vi "daqReadEtlSegment.vi"() -> ()   [LabVIEW 2017]
doc: "From the DAQ card, reads into shared variables the external frame counter, the piezo monitor, and its differentiator. The acquisition is triggered by the Hamamatsu camera triggers. If daqSave is set to true, writes the values to file. \n\nThe acquisition loop stops with a daqStop (generally issued by the hamamatsuRead* VI) or, after a delay, with a generalStop."
uses:
  <vilib>/DAQmx/read.llb/DAQmx Read (Analog 1D DBL NChan 1Samp).vi
  <vilib>/DAQmx/read.llb/DAQmx Read (Digital Bool 1Line 1Point).vi
  <vilib>/DAQmx/read.llb/DAQmx Read (Counter U32 1Chan 1Samp).vi
  globalDevices.vi
  globalUtilities.vi
  <vilib>/DAQmx/miscellaneous.llb/DAQmx Fill In Error Info.vi
panel:
  out "#problems with frame cntr":u32
  out "problem with frame counter":bool
  out "data":bool
  out "success":bool
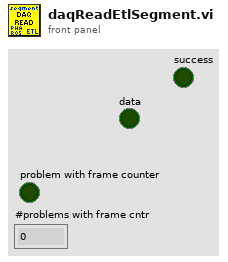
[diagram p1: front panel]
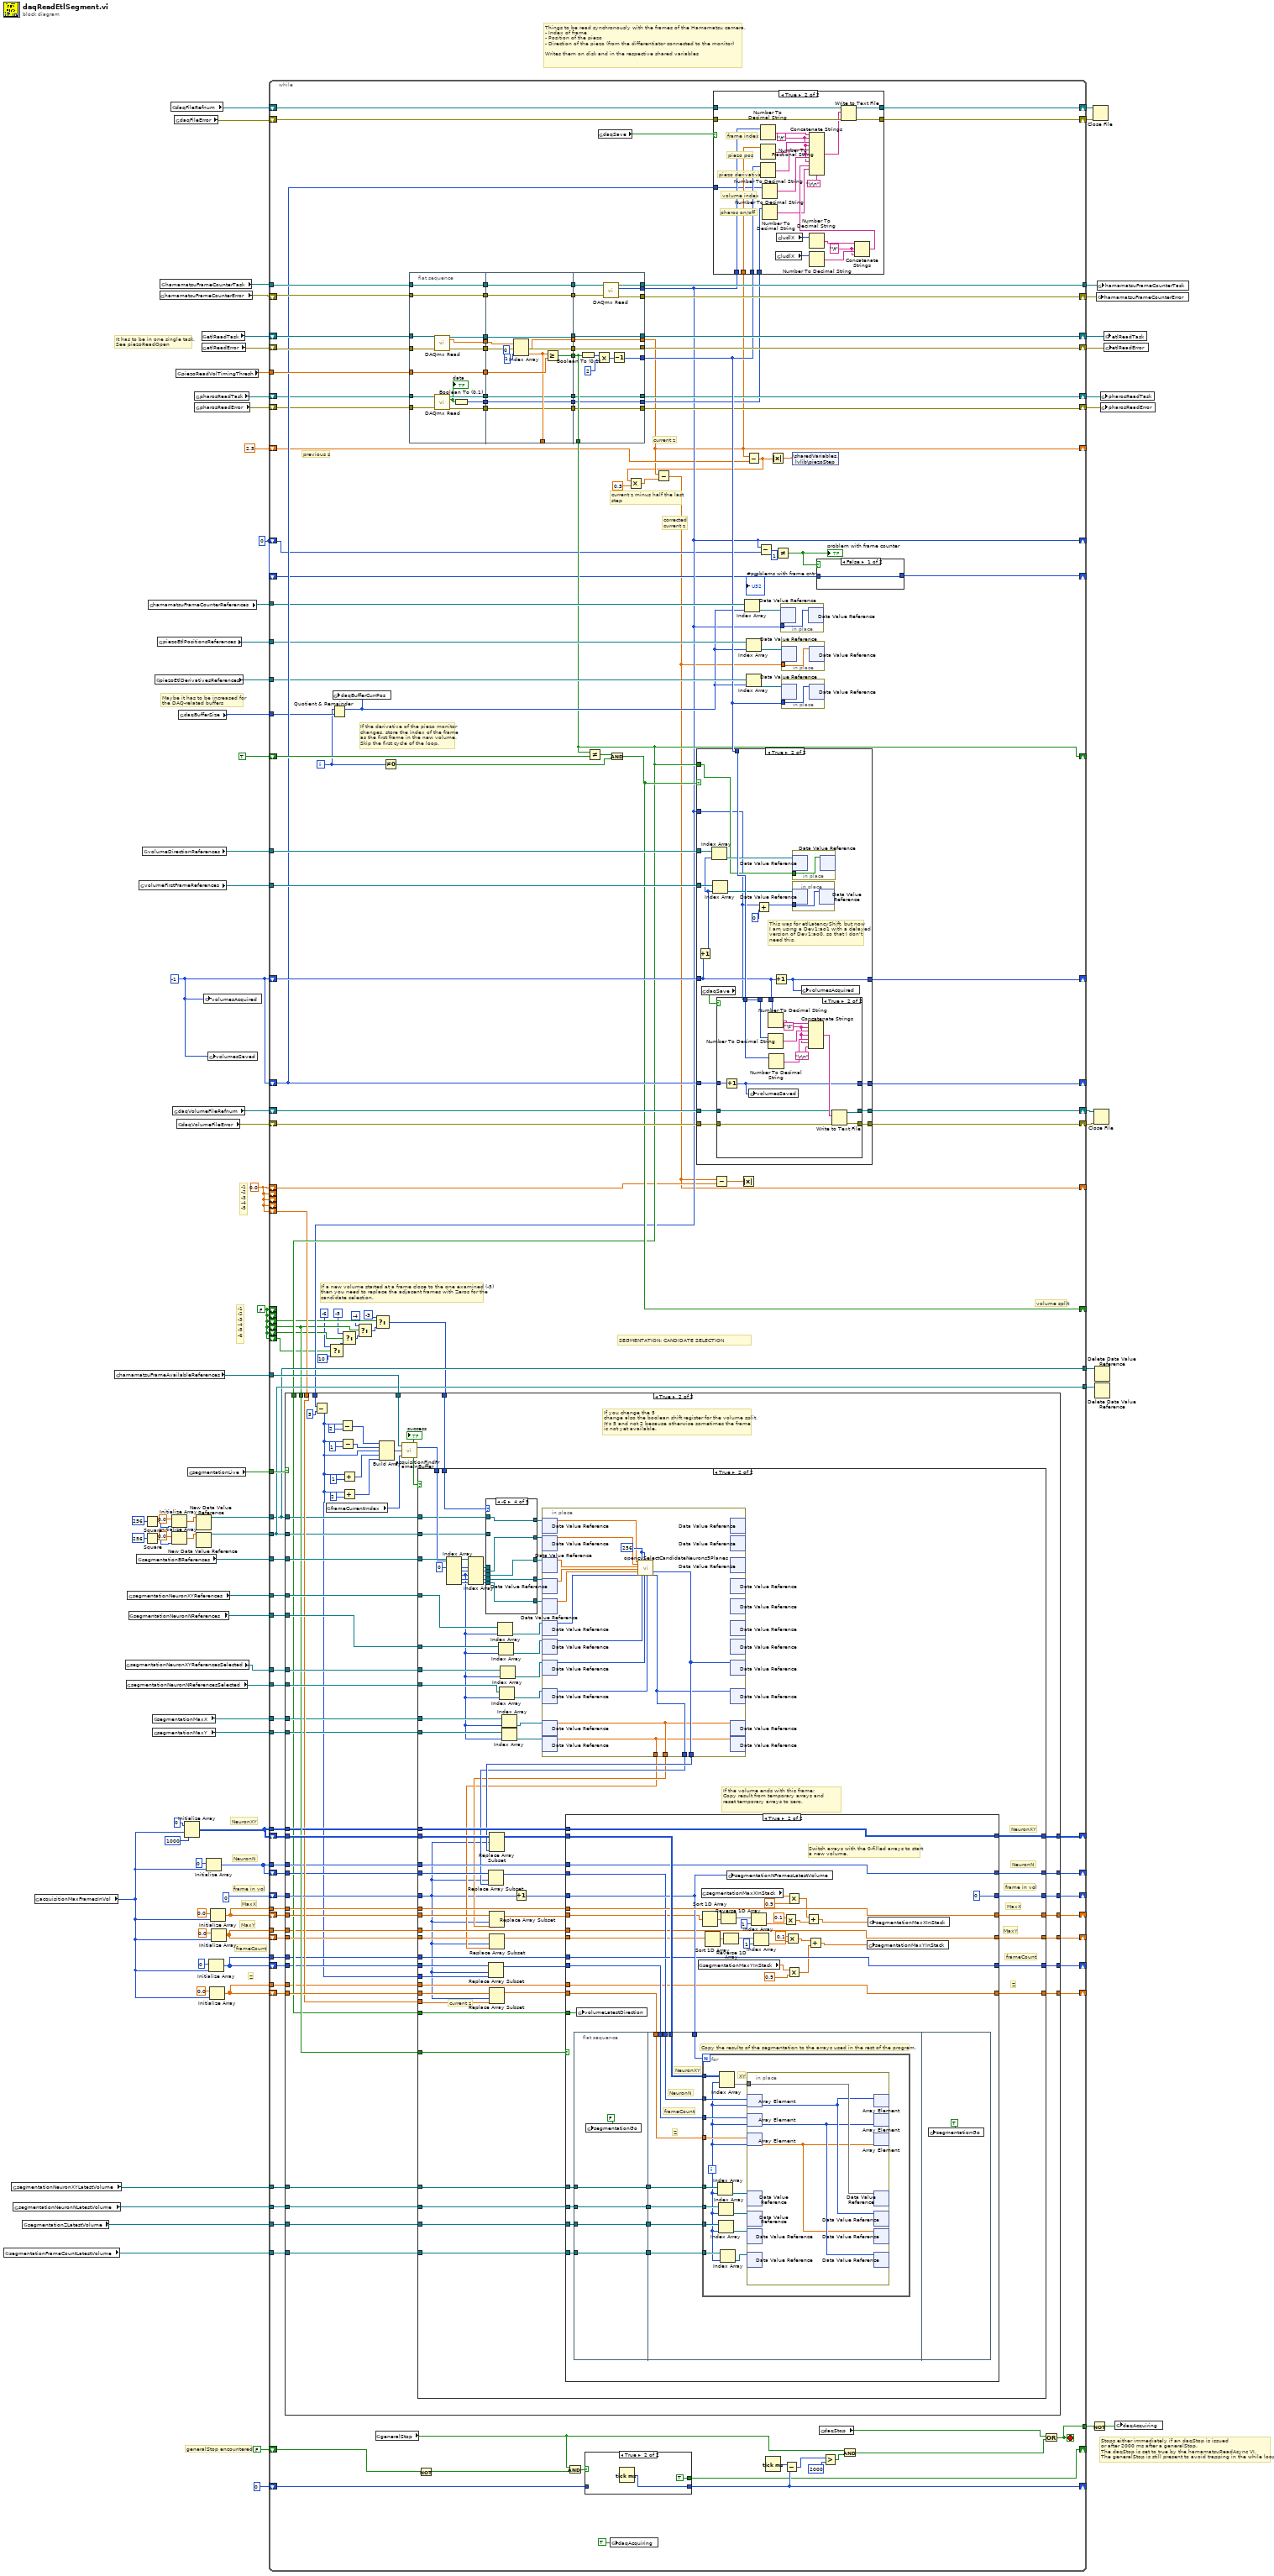
[diagram p0: block diagram]
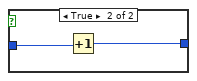
[diagram p2: hidden frame]
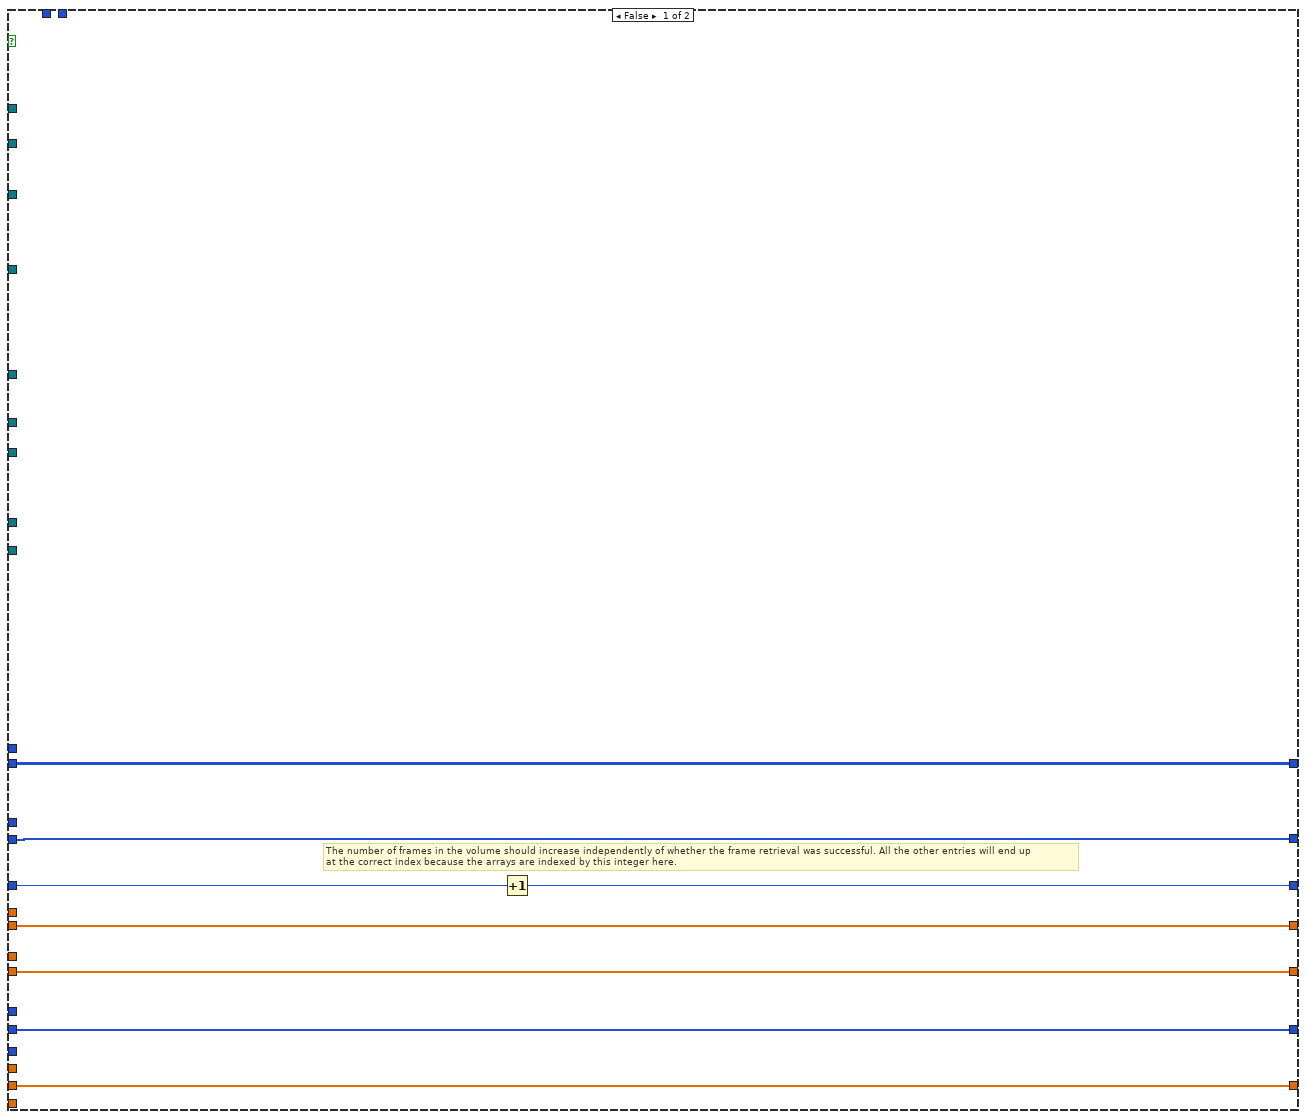
[diagram p4: hidden frame]
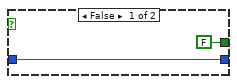
[diagram p12: hidden frame]
diagram:
  w9 = u32 0 ("data")
  w4 = FALSE
  w55 = -1
  w14 = 0.0
  # "Z"
  # "frameCount"
  # "MaxY"
  # "MaxX"
  # "frame in vol"
  # "NeuronN"
  # "NeuronXY"
  # "-1\n-2\n-3\n-4\n-5"
  # "-1\n-2\n-3\n-4\n-5\n-6"
  # "Maybe it has to be increased for\nthe DAQ-related buffers"
  # "It has to be in one single task.\nSee piezoReadOpen"
  # "generalStop encountered"
  # "Stops either immediately if an daqStop is issued\nor after 2000 ms after a generalStop.\nThe daqStop is set to true by the hamamatsuReadAsync VI.\nThe generalStop is still present to avoid trapping in the while loop."
  # "Things to be read synchronously with the frames of the Hamamatsu camera.\n- Index of frame\n- Position of the piezo\n- Direction of the piezo (from the differentiator connected to the monitor)\n\nWrites them on disk and in the respective shared variables"
  n1 = global read "globalUtilities.vi" "segmentationFrameCountLatestVolume"() -> (w8:refnum<data-value>[])
  n2 = global read "globalUtilities.vi" "segmentationNeuronXYLatestVolume"() -> (w37:refnum<data-value>[])
  n3 = global read "globalUtilities.vi" "segmentationNeuronNLatestVolume"() -> (w36:refnum<data-value>[])
  n4 = global read "globalUtilities.vi" "segmentationZLatestVolume"() -> (w33:refnum<data-value>[])
  n5 = global read "globalUtilities.vi" "acquisitionMaxFramesInVol"() -> (w6:i32)
  n6 = global read "globalDevices.vi" "hamamatsuFrameAvailableReferences"() -> (w42:refnum<data-value>[])
  n7 = global read "globalUtilities.vi" "segmentationNeuronXYReferencesSelected"() -> (w44:refnum<data-value>[])
  n8 = global read "globalUtilities.vi" "segmentationNeuronNReferencesSelected"() -> (w43:refnum<data-value>[])
  n9 = global read "globalUtilities.vi" "segmentationNeuronXYReferences"() -> (w45:refnum<data-value>[])
  n10 = global read "globalUtilities.vi" "segmentationNeuronNReferences"() -> (w47:refnum<data-value>[])
  n11 = global read "globalUtilities.vi" "segmentationBReferences"() -> (w48:refnum<data-value>[])
  n12 = global read "globalUtilities.vi" "volumeFirstFrameReferences"() -> (w56:refnum<data-value>[])
  n13 = global read "globalUtilities.vi" "volumeDirectionReferences"() -> (w57:refnum<data-value>[])
  n14 = Square(x=256) -> (x^2=w18:i32)
  n15 = Square(x=256) -> (x^2=w31:i32)
  n16 = global read "globalDevices.vi" "hamamatsuFrameCounterReferences"() -> (w52:refnum<data-value>[])
  n17 = global read "globalUtilities.vi" "segmentationMaxX"() -> (w26:refnum<data-value>[])
  n18 = global read "globalUtilities.vi" "segmentationMaxY"() -> (w25:refnum<data-value>[])
  n19 = global read "globalDevices.vi" "piezoEtlDerivativesReferences"() -> (w50:refnum<data-value>[])
  n20 = global read "globalDevices.vi" "piezoEtlPositionsReferences"() -> (w51:refnum<data-value>[])
  n21 = global read "globalDevices.vi" "hamamatsuFrameCounterError"() -> (w76:errorcluster)
  n22 = global read "globalDevices.vi" "hamamatsuFrameCounterTask"() -> (w77:refnum<k21>)
  n23 = global read "globalDevices.vi" "daqFileRefnum"() -> (w66:refnum<file>)
  n24 = Initialize Array(sgl 0.0 ("element"), w18) -> (w17:sgl[])
  n25 = Initialize Array(sgl 0.0 ("element"), w31) -> (w32:sgl[])
  n26 = global read "globalDevices.vi" "daqVolumeFileRefnum"() -> (w61:refnum<file>)
  n27 = global read "globalDevices.vi" "daqFileError"() -> (w65:errorcluster)
  n28 = global read "globalDevices.vi" "piezoReadVolTimingThresh"() -> (w72:dbl)
  n29 = global read "globalDevices.vi" "daqVolumeFileError"() -> (w60:errorcluster)
  n30 = global read "globalDevices.vi" "daqBufferSize"() -> (w49:i32)
  n31 = Initialize Array(u16 0 ("element"), w6, 1000 ("dimension size")) -> (w35:u16[][])
  n32 = global read "globalUtilities.vi" "segmentationLive"() -> (w46:bool)
  n33 = global read "globalDevices.vi" "pharosReadTask"() -> (w13:refnum<k21>)
  n34 = global read "globalDevices.vi" "pharosReadError"() -> (w12:errorcluster)
  n35 = New Data Value Reference(data value=w17) -> (data value reference=w16:refnum<data-value>)  [unwired: 1 in, 1 out]
  n36 = New Data Value Reference(data value=w32) -> (data value reference=w28:refnum<data-value>)  [unwired: 1 in, 1 out]
  n37 = global read "globalDevices.vi" "etlReadTask"() -> (w54:refnum<k21>)
  n38 = global read "globalDevices.vi" "etlReadError"() -> (w53:errorcluster)
  n39 = global write "globalUtilities.vi" "volumesAcquired"(w55) -> ()
  n40 = Initialize Array(u16 0 ("element"), w6) -> (w21:u16[])
  n41 = global write "globalUtilities.vi" "volumesSaved"(w55) -> ()
  n42 = Initialize Array(0 ("element"), w6) -> (w5:i32[])
  n43 = Initialize Array(0.0 ("element"), w6) -> (w2:dbl[])
  n44 = Initialize Array(0.0 ("element"), w6) -> (w22:dbl[])
  n45 = Initialize Array(0.0 ("element"), w6) -> (w3:dbl[])
  n46 = while {
    tunnel: w77 -> [w217]
    shift-right: [w213] -> w68
    shift-left: w76 -> [w215]
    shift-right: [w211] -> w69
    shift-left: w53 -> [w214]
    shift-right: [w208] -> w75
    shift-left: w66 -> [w209]
    shift-right: [w195] -> _
    shift-left: FALSE -> [w206]
    shift-right: [w200] -> _
    shift-left: u32 0 -> [w203]
    tunnel: w72 -> [w194]
    shift-right: [w126] -> _
    shift-left: TRUE -> [w192]
    shift-right: [w188] -> w70
    shift-left: w54 -> [w219]
    tunnel: [w187] -> w67
    shift-right: [w179] -> w64
    shift-left: w65 -> [w210]
    tunnel: [w176] -> w63
    shift-right: [w82] -> _
    shift-left: w14 -> [w87]
    shift-right: [w172] -> w58
    shift-left: w60 -> [w174]
    shift-right: [w173] -> w59
    shift-left: w61 -> [w175]
    shift-right: [w170] -> _
    shift-left: w55 -> [w171]
    tunnel: w57 -> [w169]
    tunnel: w56 -> [w168]
    shift-right: [w167] -> _
    shift-left: w55 -> [w166]
    tunnel: w52 -> [w165]
    tunnel: w51 -> [w164]
    tunnel: w50 -> [w163]
    tunnel: w49 -> [w162]
    tunnel: w48 -> [w156]
    tunnel: w47 -> [w155]
    tunnel: w46 -> [w150]
    tunnel: w45 -> [w154]
    tunnel: w44 -> [w153]
    tunnel: w43 -> [w152]
    tunnel: w42 -> [w151]
    shift-right: [w147] -> _
    shift-left: w35 -> [w149]
    shift-right: [w148] -> _
    shift-left: w4 -> [_]
    shift-left: w4 -> [_]
    shift-left: w4 -> [w102]
    shift-left: w4 -> [w99]
    shift-left: w4 -> [w97]
    shift-right: [w145] -> _
    shift-left: w21 -> [w146]
    shift-right: [w143] -> _
    shift-left: 0 -> [w144]
    tunnel: w37 -> [w142]
    tunnel: w36 -> [w141]
    tunnel: w35 -> [w140]
    shift-right: [w138] -> _
    shift-left: w2 -> [w139]
    tunnel: w33 -> [w137]
    shift-left: w14 -> [_]
    shift-left: w14 -> [_]
    shift-left: w14 -> [_]
    shift-left: w14 -> [w103]
    tunnel: w28 -> [w136]
    tunnel: [w136] -> w27
    tunnel: w26 -> [w135]
    tunnel: w25 -> [w134]
    shift-right: [w131] -> _
    shift-left: w3 -> [w132]
    shift-right: [w130] -> _
    shift-left: w22 -> [w133]
    tunnel: w22 -> [w129]
    tunnel: w21 -> [w128]
    tunnel: w16 -> [w127]
    tunnel: [w127] -> w15
    shift-right: [w121] -> w11
    shift-left: w13 -> [w125]
    shift-right: [w118] -> w10
    shift-left: w12 -> [w124]
    shift-right: [w114] -> _
    shift-left: w9 -> [w113]
    shift-right: [w109] -> _
    shift-left: w9 -> [w108]
    shift-right: [w106] -> _
    shift-left: w5 -> [w107]
    tunnel: w5 -> [w105]
    tunnel: w8 -> [w104]
    shift-left: w4 -> [w94]
    tunnel: w3 -> [w90]
    tunnel: w2 -> [w89]
    shift-right: [w83] -> _
    shift-left: 2.5 ("Waveform") -> [w84]
    i -> [w85]
    stop <- w176 stop-if-true
    # "corrected\ncurrent z"
    # "current z"
    # "current z minus half the last\nstep"
    # "previous z"
    # "volume split"
    # "SEGMENTATION: CANDIDATE SELECTION"
    # "If a new volume started at a frame close to the one examined (-5)\nthen you need to replace the adjacent frames with Zeros for the\ncandidate selection."
    # "If the derivative of the piezo monitor\nchanges, store the index of the frame\nas the first frame in the new volume.\nSkip the first cycle of the loop."
    n47 = Select(t=-6, s=w94, f=10) -> (s? t:f=w92:i32)
    n48 = Quotient & Remainder(x=w85, y=w162) -> (x-y*floor(x/y)=w157:i32)  [unwired: 1 out]
    n49 = global write "globalDevices.vi" "daqBufferCurrPos"(w157) -> ()
    n50 = Select(t=-5, s=w97, f=w92) -> (s? t:f=w95:i32)
    n51 = Select(t=-4, s=w99, f=w95) -> (s? t:f=w100:i32)
    n52 = Select(t=-3, s=w102, f=w100) -> (s? t:f=w91:i32)
    n53 = case shown="True" w150 {
      tunnel: w156 -> [_ w282]
      tunnel: w114 -> [_ w281]
      tunnel: w155 -> [_ w275]
      tunnel: w154 -> [_ w274]
      tunnel: w153 -> [_ w273]
      tunnel: w152 -> [_ w272]
      tunnel: w151 -> [_ w266]
      tunnel: w149 -> [w229 w263]
      tunnel: w99 -> [_ w262]
      tunnel: [w229 w261] -> w147
      tunnel: w146 -> [w228 w241]
      tunnel: [w228 w260] -> w145
      tunnel: w144 -> [w227 w259]
      tunnel: [w227 w258] -> w143
      tunnel: w142 -> [_ w257]
      tunnel: w141 -> [_ w256]
      tunnel: w140 -> [_ w255]
      tunnel: w103 -> [_ w252]
      tunnel: w139 -> [w226 w254]
      tunnel: [w226 w253] -> w138
      tunnel: w137 -> [_ w251]
      tunnel: w136 -> [_ w250]
      tunnel: w135 -> [_ w249]
      tunnel: w134 -> [_ w248]
      tunnel: w133 -> [w225 w247]
      tunnel: w132 -> [w224 w246]
      tunnel: [w224 w245] -> w131
      tunnel: [w225 w244] -> w130
      tunnel: w129 -> [_ w243]
      tunnel: w128 -> [_ w242]
      tunnel: w127 -> [_ w240]
      tunnel: w126 -> [_ w238]
      tunnel: w107 -> [w223 w237]
      tunnel: [w223 w236] -> w106
      tunnel: w105 -> [_ w235]
      tunnel: w104 -> [_ w234]
      tunnel: w91 -> [_ w233]
      tunnel: w90 -> [_ w232]
      tunnel: w89 -> [_ w230]
      frame False {
      }
      frame True {
        # "If you change the 5\nchange also the boolean shift register for the volume split.\nIt's 5 and not 2 because otherwise sometimes the frame \nis not yet available."
        n54 = Subtract(x=w281, y=u32 5) -> (x-y=w231:u32)
        n55 = global read "globalUtilities.vi" "frameCurrentIndex"() -> (w265:i32)
        n56 = Subtract(x=w231, y=u32 2) -> (x-y=w271:u32)
        n57 = Subtract(x=w231, y=u32 1) -> (x-y=w270:u32)
        n58 = Add(x=w231, y=u32 1) -> (x+y=w269:u32)
        n59 = Add(x=w231, y=u32 2) -> (x+y=w268:u32)
        n60 = Build Array(w271, w270, w231, w269, w268) -> (w267:u32[])
        n61 = call "acquisitionFindFrameInBuffer.vi"("startBufferIndex"=w265, "frameCounts"=w267, "hamamatsuFrameAvailableReferences"=w266) -> ("success"=w239:bool, "frameIndices"=w264:i32[])
        "success" <- w239
        n62 = case shown="True" w239 {
          tunnel: w282 -> [_ w362]
          tunnel: w275 -> [_ w361]
          tunnel: w274 -> [_ w360]
          tunnel: w273 -> [_ w357]
          tunnel: w272 -> [_ w356]
          tunnel: w264 -> [_ w353]
          tunnel: w263 -> [w290 w312]
          tunnel: w262 -> [_ w347]
          tunnel: [w290 w345] -> w261
          tunnel: w241 -> [w289 w309]
          tunnel: [w289 w344] -> w260
          tunnel: w259 -> [w288 w292]
          tunnel: [w283 w346] -> w258
          tunnel: w257 -> [_ w343]
          tunnel: w256 -> [_ w342]
          tunnel: w255 -> [_ w341]
          tunnel: w254 -> [w287 w294]
          tunnel: [w287 w340] -> w253
          tunnel: w252 -> [_ w291]
          tunnel: w251 -> [_ w339]
          tunnel: w250 -> [_ w325]
          tunnel: w249 -> [_ w338]
          tunnel: w248 -> [_ w337]
          tunnel: w247 -> [w286 w305]
          tunnel: w246 -> [w285 w301]
          tunnel: [w285 w334] -> w245
          tunnel: [w286 w333] -> w244
          tunnel: w243 -> [_ w332]
          tunnel: w242 -> [_ w331]
          tunnel: w240 -> [_ w323]
          tunnel: w238 -> [_ w317]
          tunnel: w237 -> [w284 w298]
          tunnel: [w284 w316] -> w236
          tunnel: w235 -> [_ w315]
          tunnel: w234 -> [_ w314]
          tunnel: w233 -> [_ w313]
          tunnel: w232 -> [_ w302]
          tunnel: w231 -> [_ w296]
          tunnel: w230 -> [_ w295]
          frame False {
            # "The number of frames in the volume should increase independently of whether the frame retrieval was successful. All the other entries will end up\nat the correct index because the arrays are indexed by this integer here."
            n63 = Increment(x=w288) -> (x+1=w283:i32)
          }
          frame True {
            # "current z"
            # "If the volume ends with this frame:\nCopy result from temporary arrays and\nreset temporary arrays to zero."
            # "frameCount"
            # "Z"
            # "frame in vol"
            # "MaxY"
            # "MaxX"
            # "NeuronN"
            # "NeuronXY"
            n64 = Index Array(array=w353, index #1=0 ("index")) -> (element #1=w351:i32, element #2=w350:i32, element #3=w318:i32, element #4=w349:i32, element #5=w348:i32)  [unwired: 4 in]
            n65 = Index Array(array=w362, index #1=w351, index #2=w350, index #3=w318, index #4=w349, index #5=w348) -> (element #1=w330:refnum<data-value>, element #2=w329:refnum<data-value>, element #3=w328:refnum<data-value>, element #4=w327:refnum<data-value>, element #5=w326:refnum<data-value>)
            n66 = case shown="-6" w313 {
              tunnel: w330 -> [w367 w372 _ _ w387]
              tunnel: w329 -> [w366 w371 _ w381 w386]
              tunnel: w328 -> [w365 w370 w377 w380 w385]
              tunnel: w327 -> [w364 _ w374 w379 w384]
              tunnel: w326 -> [_ _ w373 w378 w383]
              tunnel: w325 -> [w363 w369 w375 _ _]
              tunnel: [w365 w370 w377 w380 w385] -> w324
              tunnel: w323 -> [_ w368 w376 w382 _]
              tunnel: [w367 w372 w376 w382 w387] -> w322
              tunnel: [w366 w371 w375 w381 w386] -> w321
              tunnel: [w364 w368 w374 w379 w384] -> w320
              tunnel: [w363 w369 w373 w378 w383] -> w319
              frame -3 {
              }
              frame -4 {
              }
              frame -5 {
              }
              frame -6 {
              }
              frame 10, Default {
              }
            }
            n67 = Replace Array Subset(array=w298, new element=w296, index=w292) -> (w297:i32[])
            n68 = Replace Array Subset(array=w294, new element=w291, index=w292) -> (w293:dbl[])
            n69 = Index Array(array=w360, index=w318) -> (element=w359:refnum<data-value>)
            n70 = Index Array(array=w361, index=w318) -> (element=w358:refnum<data-value>)
            n71 = Index Array(array=w356, index=w318) -> (element=w354:refnum<data-value>)
            n72 = Index Array(array=w357, index=w318) -> (element=w355:refnum<data-value>)
            n73 = Index Array(array=w338, index=w318) -> (element=w335:refnum<data-value>)
            n74 = Index Array(array=w337, index=w318) -> (element=w336:refnum<data-value>)
            n75 = Increment(x=w292) -> (x+1=w306:i32)
            n76 = in-place {
              in-place-border: [w477] -> w310
              in-place-border: [w476] -> w308
              in-place-border: [w475] -> w303
              in-place-border: [w474] -> w299
              w473 = 256 ("sizeBx")
              n77 = in-place-dvr #1(w322) -> (w471:sgl[])  [unwired: 1 out]
              n78 = in-place-dvr #2(w321) -> (w484:sgl[])  [unwired: 1 out]
              n79 = in-place-dvr #3(w324) -> (w483:sgl[])  [unwired: 1 out]
              n80 = in-place-dvr #4(w320) -> (w482:sgl[])  [unwired: 1 out]
              n81 = in-place-dvr #5(w319) -> (w481:sgl[])  [unwired: 1 out]
              n82 = in-place-dvr #6(w359) -> (w480:u16[])  [unwired: 1 out]
              n83 = in-place-dvr #7(w358) -> (w472:u16)  [unwired: 1 out]
              n84 = in-place-dvr #8(w355) -> (w479:u16[])  [unwired: 1 out]
              n85 = in-place-dvr #9(w354) -> (w478:u16)  [unwired: 1 out]
              n86 = in-place-dvr #10(w335) -> (w475:dbl)  [unwired: 1 out]
              n87 = in-place-dvr #11(w336) -> (w474:dbl)  [unwired: 1 out]
              n88 = call "opencvSelectCandidateNeurons5Planes.vi"("ArrB0"=w471, "ArrB1"=w484, "ArrB2"=w483, "ArrB3"=w482, "ArrB4"=w481, "NeuronXYin"=w480, "sizeBx"=w473, "NeuronNin"=w472, "sizeBy"=w473, "NeuronXYout"=w479, "NeuronNout"=w478) -> ("NeuronXYout out"=w477:u16[], "NeuronNout out"=w476:u16)  [unwired: 3 in, 4 out]
              n89 = in-place-dvr #1() -> ()  [unwired: 1 in, 2 out]
              n90 = in-place-dvr #2() -> ()  [unwired: 1 in, 2 out]
              n91 = in-place-dvr #3() -> ()  [unwired: 1 in, 2 out]
              n92 = in-place-dvr #4() -> ()  [unwired: 1 in, 2 out]
              n93 = in-place-dvr #5() -> ()  [unwired: 1 in, 2 out]
              n94 = in-place-dvr #6() -> ()  [unwired: 1 in, 2 out]
              n95 = in-place-dvr #7() -> ()  [unwired: 1 in, 2 out]
              n96 = in-place-dvr #8(w477) -> ()  [unwired: 2 out]
              n97 = in-place-dvr #9(w476) -> ()  [unwired: 2 out]
              n98 = in-place-dvr #10(w475) -> ()  [unwired: 2 out]
              n99 = in-place-dvr #11(w474) -> ()  [unwired: 2 out]
            }
            n100 = Replace Array Subset(array=w309, new element=w308, index=w292) -> (w307:u16[])
            n101 = Replace Array Subset(array=w312, new element=w310, index (row)=w292) -> (w311:u16[][])  [unwired: 1 in]
            n102 = Replace Array Subset(array=w305, new element=w303, index=w292) -> (w304:dbl[])
            n103 = Replace Array Subset(array=w301, new element=w299, index=w292) -> (w300:dbl[])
            n104 = case shown="True" w347 {
              tunnel: w311 -> [w393 w434]
              tunnel: w306 -> [w394 w428]
              tunnel: [w394 0] -> w346
              tunnel: [w393 w433] -> w345
              tunnel: [w392 w429] -> w344
              tunnel: w343 -> [_ w436]
              tunnel: w342 -> [_ w435]
              tunnel: w341 -> [_ w433]
              tunnel: w293 -> [w388 w431]
              tunnel: [w388 w421] -> w340
              tunnel: w339 -> [_ w432]
              tunnel: w304 -> [w391 w416]
              tunnel: w300 -> [w390 w409]
              tunnel: [w390 w422] -> w334
              tunnel: [w391 w430] -> w333
              tunnel: w332 -> [_ w430]
              tunnel: w331 -> [_ w429]
              tunnel: w317 -> [_ w427]
              tunnel: w297 -> [w389 w424]
              tunnel: [w389 w426] -> w316
              tunnel: w315 -> [_ w426]
              tunnel: w314 -> [_ w425]
              tunnel: w307 -> [w392 w423]
              tunnel: w302 -> [_ w422]
              tunnel: w295 -> [_ w421]
              frame False {
              }
              frame True {
                # "Switch arrays with the 0-filled arrays to start\na new volume."
                n105 = flat-sequence {
                  tunnel: w425 -> [w439]
                  tunnel: w432 -> [w440]
                  tunnel: w435 -> [w441]
                  tunnel: w436 -> [w442]
                  tunnel: [w442] -> w420
                  tunnel: [w441] -> w419
                  tunnel: [w440] -> w418
                  tunnel: [w439] -> w417
                  tunnel: w434 -> [w449]
                  tunnel: w431 -> [w447]
                  tunnel: w428 -> [w446]
                  tunnel: w424 -> [w444]
                  tunnel: w423 -> [w443]
                  tunnel: w420 -> [w451]
                  tunnel: w419 -> [w450]
                  tunnel: w418 -> [w448]
                  tunnel: w417 -> [w445]
                  frame #0 {
                    n106 = global write "globalUtilities.vi" "segmentationGo"(FALSE ("segmentationGo")) -> ()
                  }
                  frame #1 {
                    # "Z"
                    # "frameCount"
                    # "NeuronXY"
                    # "NeuronN"
                    # "Copy the results of the segmentation to the arrays used in the rest of the program."
                    n107 = for {
                      N: w446 -> [_]
                      tunnel: w451 -> [w465]
                      tunnel: w450 -> [w464]
                      tunnel: w449 -> [w460]
                      tunnel: w448 -> [w458]
                      tunnel: w445 -> [w455]
                      tunnel: w447 -> [w456]
                      tunnel: w443 -> [w463]
                      tunnel: w444 -> [w453]
                      i -> [w452]
                      # "XY"
                      n108 = Index Array(array=w465, index=w452) -> (element=w462:refnum<data-value>)
                      n109 = Index Array(array=w464, index=w452) -> (element=w461:refnum<data-value>)
                      n110 = Index Array(array=w458, index=w452) -> (element=w457:refnum<data-value>)
                      n111 = Index Array(array=w460, index (row)=w452) -> (element=w459:u16[])  [unwired: 1 in]
                      n112 = Index Array(array=w455, index=w452) -> (element=w454:refnum<data-value>)
                      n113 = in-place {
                        in-place-border: w459 -> [w469]
                        n114 = in-place-array #12(w463, w452) -> (w468:u16)
                        n115 = in-place-array #13(w453, w452) -> (w467:i32)
                        n116 = in-place-array #14(w456, w452) -> (w466:dbl)
                        n117 = in-place-dvr #15(w462) -> ()  [unwired: 2 out]
                        n118 = in-place-dvr #16(w461) -> ()  [unwired: 2 out]
                        n119 = in-place-dvr #17(w457) -> ()  [unwired: 2 out]
                        n120 = in-place-dvr #18(w454) -> ()  [unwired: 2 out]
                        n121 = in-place-array #12(w468) -> ()  [unwired: 2 out]
                        n122 = in-place-array #13(w467) -> ()  [unwired: 2 out]
                        n123 = in-place-array #14(w466) -> ()  [unwired: 2 out]
                        n124 = in-place-dvr #15(w469) -> ()  [unwired: 2 out]
                        n125 = in-place-dvr #16(w468) -> ()  [unwired: 2 out]
                        n126 = in-place-dvr #17(w466) -> ()  [unwired: 2 out]
                        n127 = in-place-dvr #18(w467) -> ()  [unwired: 2 out]
                      }
                    }
                  }
                  frame #2 {
                    n128 = global write "globalUtilities.vi" "segmentationGo"(TRUE ("segmentationGo")) -> ()
                  }
                }
                n129 = global write "globalUtilities.vi" "volumeLatestDirection"(w427) -> ()
                n130 = global read "globalUtilities.vi" "segmentationMaxYInStack"() -> (w405:dbl)
                n131 = global read "globalUtilities.vi" "segmentationMaxXInStack"() -> (w408:dbl)
                n132 = Sort 1D Array(array=w416) -> (sorted array=w415:dbl[])
                n133 = Sort 1D Array(array=w409) -> (sorted array=w412:dbl[])
                n134 = Reverse 1D Array(array=w415) -> (reversed array=w414:dbl[])
                n135 = Reverse 1D Array(array=w412) -> (reversed array=w411:dbl[])
                n136 = global write "globalUtilities.vi" "segmentationNFramesLatestVolume"(w428) -> ()
                n137 = Index Array(array=w414, index=1) -> (element=w404:dbl)
                n138 = Index Array(array=w411, index=1) -> (element=w398:dbl)
                n139 = Multiply(x=0.1, y=w404) -> (x*y=w402:dbl)
                n140 = Multiply(x=0.1, y=w398) -> (x*y=w397:dbl)
                n141 = Multiply(x=w408, y=0.9) -> (x*y=w401:dbl)
                n142 = Multiply(x=w405, y=0.9) -> (x*y=w396:dbl)
                n143 = Add(x=w401, y=w402) -> (x+y=w400:dbl)
                n144 = Add(x=w397, y=w396) -> (x+y=w395:dbl)
                n145 = global write "globalUtilities.vi" "segmentationMaxYInStack"(w395) -> ()
                n146 = global write "globalUtilities.vi" "segmentationMaxXInStack"(w400) -> ()
              }
            }
          }
        }
      }
    }
    n147 = global read "globalUtilities.vi" "generalStop"() -> (w202:bool)
    n148 = Not Equal To 0?(x=w85) -> (x != 0?=w190:bool)
    n149 = flat-sequence {
      tunnel: w194 -> [w571]
      tunnel: w215 -> [w572]
      tunnel: w214 -> [w569]
      tunnel: w217 -> [w573]
      tunnel: w219 -> [w570]
      tunnel: [w573] -> w186
      tunnel: [w572] -> w185
      tunnel: [w571] -> w184
      tunnel: [w568] -> w183
      tunnel: [w567] -> w182
      tunnel: [w566] -> w180
      tunnel: w125 -> [w565]
      tunnel: w124 -> [w564]
      tunnel: [w563] -> w122
      tunnel: [w562] -> w119
      tunnel: [w560] -> w116
      tunnel: [w587] -> w218
      tunnel: [w586] -> w216
      tunnel: [w582] -> w212
      tunnel: [w584] -> w193
      tunnel: [w577] -> _
      tunnel: [w583] -> w189
      tunnel: w186 -> [w587]
      tunnel: w185 -> [w586]
      tunnel: w184 -> [w585]
      tunnel: w183 -> [w583]
      tunnel: w182 -> [w581]
      tunnel: [w578] -> w181
      tunnel: w180 -> [w582]
      tunnel: [w576] -> w123
      tunnel: w122 -> [w576]
      tunnel: [w575] -> w120
      tunnel: w119 -> [w575]
      tunnel: [w574] -> w117
      tunnel: w116 -> [w574]
      tunnel: w218 -> [w603]
      tunnel: w216 -> [w602]
      tunnel: [w601] -> w83
      tunnel: [w600] -> w114
      tunnel: [w599] -> w213
      tunnel: [w598] -> w211
      tunnel: w212 -> [w598]
      tunnel: w193 -> [w593]
      tunnel: [w594] -> w158
      tunnel: [w593] -> w126
      tunnel: w189 -> [w592]
      tunnel: [w592] -> w188
      tunnel: [w591] -> w187
      tunnel: w181 -> [w601]
      tunnel: [w590] -> w121
      tunnel: w123 -> [w590]
      tunnel: [w589] -> w118
      tunnel: w120 -> [w589]
      tunnel: [w588] -> w115
      tunnel: w117 -> [w588]
      frame #0 {
        n150 = call-poly <vilib>:"DAQmx Read.vi"("task/channels in"=w570, "error in"=w569) -> ("task out"=w568:refnum<k21>, "data"=w567:dbl[], "error out"=w566:errorcluster)  [unwired: 11 in]
        n151 = call-poly <vilib>:"DAQmx Read.vi"("task/channels in"=w565, "error in"=w564) -> ("task out"=w563:refnum<k21>, "data"=w561:bool, "error out"=w562:errorcluster)  [unwired: 11 in]
        "data" <- w561
        n152 = Boolean To (0,1)(Boolean=w561) -> (0, 1=w560:i16)
      }
      frame #1 {
        n153 = Index Array(array=w581, index #1=0 ("index"), index #2=1 ("index")) -> (element #1=w578:dbl, element #2=w577:dbl)
        n154 = Greater Or Equal?(x=w577, y=w585) -> (x >= y?=w584:bool)
      }
      frame #2 {
        n155 = Boolean To (0,1)(Boolean=w593) -> (0, 1=w597:i16)
        n156 = Multiply(x=w597, y=i16 2) -> (x*y=w595:i16)
        n157 = call-poly <vilib>:"DAQmx Read.vi"("task/channels in"=w603, "error in"=w602) -> ("task out"=w591:refnum<k21>, "data"=w600:u32, "error out"=w599:errorcluster)  [unwired: 11 in]
        n158 = Decrement(x=w595) -> (x-1=w594:i16)
      }
    }
    n159 = Not(x=w206) -> (.not. x?=w204:bool)
    n160 = And(x=w202, y=w204) -> (x .and. y?=w205:bool)
    n161 = case shown="True" w205 {
      tunnel: w203 -> [w532 _]
      tunnel: [w532 w534] -> w200
      tunnel: [FALSE TRUE] -> w195
      frame False {
      }
      frame True {
        n162 = Tick Count (ms)() -> (millisecond timer value=w534:u32)
      }
    }
    n163 = Not Equal?(x=w126, y=w192) -> (x != y?=w191:bool)
    n164 = global read "globalUtilities.vi" "daqSave"() -> (w207:bool)
    n165 = And(x=w191, y=w190) -> (x .and. y?=w148:bool)
    n166 = global write "globalUtilities.vi" "daqAcquiring"(TRUE ("daqAcquiring")) -> ()
    n167 = case shown="True" w148 {
      tunnel: w114 -> [_ w497]
      tunnel: w126 -> [_ w501]
      tunnel: w175 -> [w490 w509]
      tunnel: w174 -> [w489 w508]
      tunnel: [w490 w507] -> w173
      tunnel: [w489 w506] -> w172
      tunnel: w171 -> [w491 w499]
      tunnel: [w491 w504] -> w170
      tunnel: w158 -> [_ w505]
      tunnel: w169 -> [_ w503]
      tunnel: w168 -> [_ w500]
      tunnel: w166 -> [w488 w495]
      tunnel: [w488 w494] -> w167
      frame False {
      }
      frame True {
        # "This was for etlLatencyShift, but now\nI am using a Dev1:ao1 with a delayed \nversion of Dev1:ao0, so that I don't \nneed this."
        n168 = Increment(x=w499) -> (x+1=w496:i32)
        n169 = global read "globalUtilities.vi" "daqSave"() -> (w510:bool)
        n170 = Index Array(array=w503, index=w496) -> (element=w502:refnum<data-value>)
        n171 = Index Array(array=w500, index=w496) -> (element=w498:refnum<data-value>)
        n172 = case shown="True" w510 {
          tunnel: w509 -> [w515 w521]
          tunnel: w508 -> [w514 w520]
          tunnel: [w515 w519] -> w507
          tunnel: [w514 w518] -> w506
          tunnel: w499 -> [_ w530]
          tunnel: w497 -> [_ w529]
          tunnel: w505 -> [_ w528]
          tunnel: w495 -> [w513 w517]
          tunnel: [w513 w516] -> w494
          frame False {
          }
          frame True {
            w524 = "\t"
            n173 = Increment(x=w517) -> (x+1=w516:i32)
            n174 = global write "globalUtilities.vi" "volumesSaved"(w516) -> ()
            n175 = Number To Decimal String(number=w530) -> (decimal integer string=w527:string)  [unwired: 1 in]
            n176 = Number To Decimal String(number=w529) -> (decimal integer string=w526:string)  [unwired: 1 in]
            n177 = Number To Decimal String(number=w528) -> (decimal integer string=w525:string)  [unwired: 1 in]
            n178 = Concatenate Strings(w527, w524, w526, w524, w525, w524, "\r\n") -> (w522:string)
            n179 = Write to Text File(file (use dialog)=w521, text=w522, error in=w520) -> (refnum out=w519:refnum<file>, error out=w518:errorcluster)  [unwired: 1 in, 1 out]
          }
        }
        n180 = Add(x=w497, y=u32 0) -> (x+y=w493:u32)
        n181 = Increment(x=w499) -> (x+1=w504:i32)
        n182 = in-place {
          in-place-border: w501 -> [w512]
          n183 = in-place-dvr #19(w502) -> ()  [unwired: 2 out]
          n184 = in-place-dvr #19(w512) -> ()  [unwired: 2 out]
        }
        n185 = in-place {
          in-place-border: w493 -> [w511]
          n186 = in-place-dvr #20(w498) -> ()  [unwired: 2 out]
          n187 = in-place-dvr #20(w511) -> ()  [unwired: 2 out]
        }
        n188 = global write "globalUtilities.vi" "volumesAcquired"(w504) -> ()
      }
    }
    n189 = case shown="True" w207 {
      tunnel: w210 -> [w535 w557]
      tunnel: w209 -> [w536 w555]
      tunnel: [w536 w554] -> w208
      tunnel: [w535 w553] -> w179
      tunnel: w114 -> [_ w552]
      tunnel: w83 -> [_ w551]
      tunnel: w158 -> [_ w549]
      tunnel: w166 -> [_ w548]
      tunnel: w115 -> [_ w537]
      frame False {
      }
      frame True {
        w542 = "\t" ("string")
        w541 = "\t"
        # "pharos on/off"
        # "volume index"
        # "piezo derivative"
        # "piezo pos"
        # "frame index"
        n190 = Number To Decimal String(number=w552) -> (decimal integer string=w559:string)  [unwired: 1 in]
        n191 = Number To Fractional String(number=w551) -> (F-format string=w558:string)  [unwired: 3 in]
        n192 = Number To Decimal String(number=w549) -> (decimal integer string=w550:string)  [unwired: 1 in]
        n193 = Number To Decimal String(number=w548) -> (decimal integer string=w547:string)  [unwired: 1 in]
        n194 = Number To Decimal String(number=w537) -> (decimal integer string=w538:string)  [unwired: 1 in]
        n195 = global read "globalDevices.vi" "ludlX"() -> (w543:i32)
        n196 = global read "globalDevices.vi" "ludlX"() -> (w544:i32)
        n197 = Number To Decimal String(number=w544) -> (decimal integer string=w545:string)  [unwired: 1 in]
        n198 = Number To Decimal String(number=w543) -> (decimal integer string=w546:string)  [unwired: 1 in]
        n199 = Concatenate Strings(w545, w542, w546, w542) -> (w540:string)
        n200 = Concatenate Strings(w559, w541, w558, w541, w550, w541, w547, w541, w540, w538, "\r\n") -> (w556:string)
        n201 = Write to Text File(file (use dialog)=w555, text=w556, error in=w557) -> (refnum out=w554:refnum<file>, error out=w553:errorcluster)  [unwired: 1 in, 1 out]
      }
    }
    n202 = Index Array(array=w165, index=w157) -> (element=w161:refnum<data-value>)
    n203 = Subtract(x=w83, y=w84) -> (x-y=w78:dbl)
    n204 = Multiply(x=w78, y=0.5) -> (x*y=w79:dbl)
    n205 = Subtract(x=w83, y=w79) -> (x-y=w82:dbl)
    n206 = Subtract(x=w82, y=w87) -> (x-y=w86:dbl)
    n207 = Absolute Value(x=w86) -> ()  [unwired: 1 out]
    n208 = Index Array(array=w164, index=w157) -> (element=w160:refnum<data-value>)
    n209 = Index Array(array=w163, index=w157) -> (element=w159:refnum<data-value>)
    n210 = Subtract(x=w114, y=w113) -> (x-y=w112:u32)
    n211 = Tick Count (ms)() -> (millisecond timer value=w201:u32)
    n212 = Absolute Value(x=w78) -> (abs(x)=w81:dbl)
    n213 = Not Equal?(x=w112, y=u32 1) -> (x != y?=w110:bool)
    "problem with frame counter" <- w110
    n214 = in-place {
      in-place-border: w114 -> [w487]
      n215 = in-place-dvr #21(w161) -> ()  [unwired: 2 out]
      n216 = in-place-dvr #21(w487) -> ()  [unwired: 2 out]
    }
    n217 = in-place {
      in-place-border: w82 -> [w486]
      n218 = in-place-dvr #22(w160) -> ()  [unwired: 2 out]
      n219 = in-place-dvr #22(w486) -> ()  [unwired: 2 out]
    }
    n220 = in-place {
      in-place-border: w158 -> [w485]
      n221 = in-place-dvr #23(w159) -> ()  [unwired: 2 out]
      n222 = in-place-dvr #23(w485) -> ()  [unwired: 2 out]
    }
    n223 = Subtract(x=w201, y=w200) -> (x-y=w199:u32)
    n224 = shared-variable ".\\sharedVariables.lvlib\\piezoStep"(w81) -> ()  [unwired: 1 in, 1 out]
    n225 = case shown="False" w110 {
      tunnel: [w220 w222] -> w109
      tunnel: w108 -> [w220 w221]
      frame False {
      }
      frame True {
        n226 = Increment(x=w221) -> (x+1=w222:u32)
      }
    }
    n227 = global read "globalUtilities.vi" "daqStop"() -> (w177:bool)
    n228 = Greater?(x=w199, y=u32 2000) -> (0:w197:bool)
    n229 = And(x=w202, y=w197) -> (x .and. y?=w196:bool)
    n230 = Or(x=w177, y=w196) -> (x .or. y?=w176:bool)
    "#problems with frame cntr" <- w108
  }
  n231 = Not(x=w63) -> (.not. x?=w62:bool)
  n232 = Close File(refnum=w75, error in=w64) -> ()  [unwired: 2 out]
  n233 = Close File(refnum=w59, error in=w58) -> ()  [unwired: 2 out]
  n234 = Delete Data Value Reference(data value reference=w15) -> ()  [unwired: 1 in, 2 out]
  n235 = Delete Data Value Reference(data value reference=w27) -> ()  [unwired: 1 in, 2 out]
  n236 = global write "globalDevices.vi" "hamamatsuFrameCounterError"(w68) -> ()
  n237 = global write "globalDevices.vi" "hamamatsuFrameCounterTask"(w67) -> ()
  n238 = global write "globalDevices.vi" "pharosReadTask"(w11) -> ()
  n239 = global write "globalDevices.vi" "pharosReadError"(w10) -> ()
  n240 = global write "globalDevices.vi" "etlReadTask"(w70) -> ()
  n241 = global write "globalDevices.vi" "etlReadError"(w69) -> ()
  n242 = global write "globalUtilities.vi" "daqAcquiring"(w62) -> ()
